vi "Reserve Devices.vi"(0 "session in":refnum<k21>, 5 "devices":refnum<k21>="$DefaultDevices", 7 "reservation access (Read/Write)":i32(ring)=3 items=["Read Only"=1, "Read/Write"=3], 9 "reservation group":string, 11 "error in (no error)":errorcluster, 13 "reservation timeout (0 sec)":dbl) -> (4 "session out":refnum<k21>, 15 "error out":errorcluster)   [LabVIEW 2020, in "SLSC.lvlib"]
doc: "Reserves one or multiple devices to prevent other sessions from access the devices. You must reserve a device before using it."
uses:
  <vilib>/SLSC/SLSC.lvlib
  nislsclvapi.dll
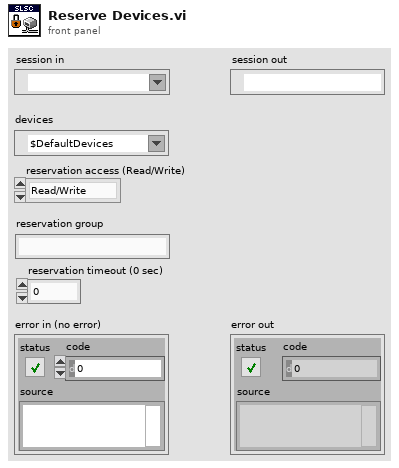
[diagram p1: front panel]
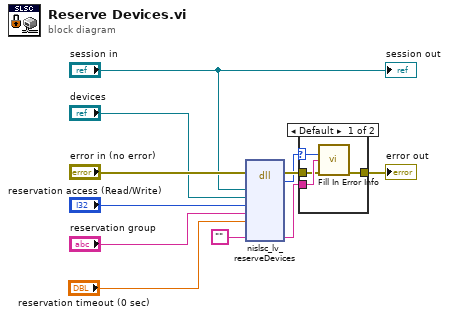
[diagram p0: block diagram]
diagram:
  n1 = dll-call lib="nislsclvapi.*" fn="nislsc_lv_reserveDevices"(error in="error in (no error)", "session"="session in", "devices"="devices", "reservationAccess"="reservation access (Read/Write)", "reservationGroup"="reservation group", "reservationTimeout"="reservation timeout (0 sec)", "extendedErrorInfo"="") -> (error out=w6:errorcluster, "return type"=w5:i32, "extendedErrorInfo"=w4:string)  [unwired: 9 in, 1 out]
  n2 = case shown="Default" w5 {
    selector: w5 -> [w15 _]
    tunnel: w4 -> [w14 _]
    tunnel: w6 -> [w13 w16]
    tunnel: [w12 w16] -> w3
    frame Default {
      n3 = call <vilib>:"Fill In Error Info.vi"("status code"=w15, "extended error info"=w14, "error in"=w13) -> ("error out"=w12:errorcluster)  [unwired: 12 in]
    }
    frame 0 {
    }
  }
  "error out" <- w3
  "session out" <- "session in"
